vi "Insert.vi"(6 "Item":T1, 9 "<JSON>name":string, 10 "JSON to Insert":string, 11 "JSON in":string) -> (1 "Inserted Item Offset":i32, 2 "Found":bool, 3 "string":string)   [LabVIEW 2015, in "JSONtext.lvlib"]
uses:
  JSONtext.lvlib
  Found Items.ctl
  Advance past whitespace.vi
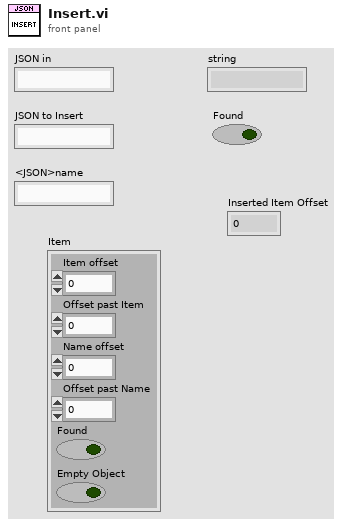
[diagram p1: front panel]
types:
  T1 = typedef "JSONtext.lvlib/Found Items.ctl" = cluster{"Item offset":i32, "Offset past Item":i32, "Name offset":i32, "Offset past Name":i32, "Found":bool, "Empty Object":bool}
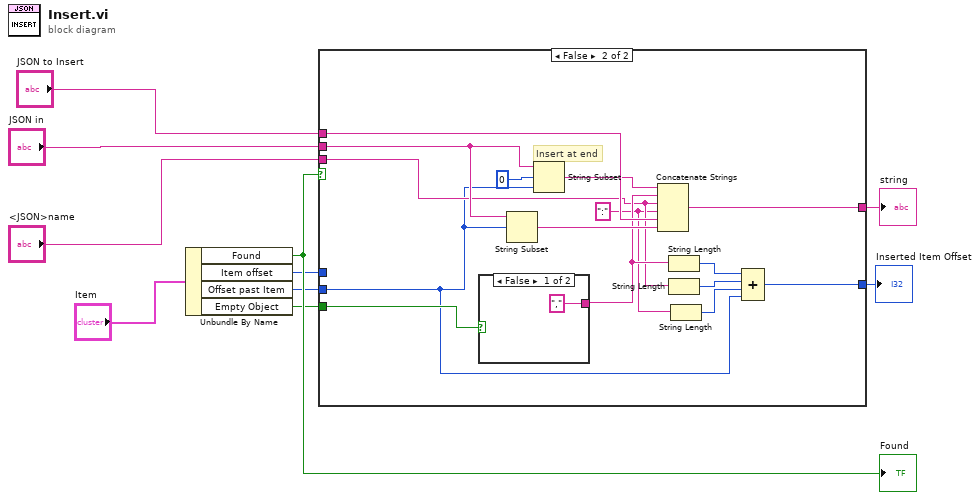
[diagram p0: block diagram]
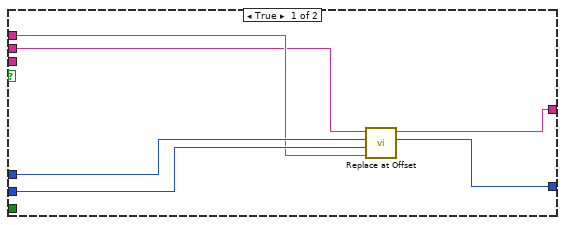
[diagram p2: hidden frame]
diagram:
  n1 = Unbundle By Name("Item") -> ("Found"=w9:bool, "Item offset"=w5:i32, "Offset past Item"=w4:i32, "Empty Object"=w3:bool)
  "Found" <- w9
  n2 = case shown="False" w9 {
    tunnel: "JSON in" -> [w12 w31]
    tunnel: "JSON to Insert" -> [w13 w30]
    tunnel: [w16 w29] -> w7
    tunnel: "<JSON>name" -> [_ w23]
    tunnel: w5 -> [w15 _]
    tunnel: w4 -> [w14 w17]
    tunnel: w3 -> [_ w25]
    tunnel: [w11 w18] -> w1
    frame True {
      n3 = call "Replace at Offset.vi"("JSON to Insert"=w13, "Offset past Item"=w14, "Item offset"=w15, "<JSON> in"=w12) -> ("Item offset"=w11:i32, "<JSON>"=w16:string)  [unwired: 6 in]
    }
    frame False {
      w22 = ":" ("string")
      # "Insert at end"
      n4 = case shown="False" w25 {
        tunnel: ["," ("string") _] -> w24
        frame False {
        }
        frame True {
        }
      }
      n5 = String Subset(string=w31, offset (0)=w17) -> (substring=w26:string)  [unwired: 1 in]
      n6 = String Subset(string=w31, offset (0)=0 ("Value start in"), length (rest)=w17) -> (substring=w27:string)
      n7 = Concatenate Strings(w27, w24, w23, w22, w30, w26) -> (w29:string)
      n8 = String Length(string=w24) -> (length=w21:i32)
      n9 = String Length(string=w23) -> (length=w20:i32)
      n10 = String Length(string=w22) -> (length=w19:i32)
      n11 = Compound Arithmetic op=ADD(w21, w20, w19, w17) -> (w18:i32)
    }
  }
  "string" <- w7
  "Inserted Item Offset" <- w1
